vi "CRYClear Main Generator Array.vi"(9 "isMain":bool, 11 "Gen Idx":i32) -> (0 "isMain out":bool)   [LabVIEW 2013]
uses:
  CRYMisc vis settings global.vi
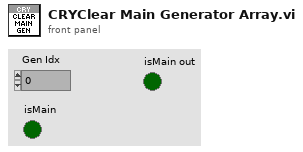
[diagram p1: front panel]
types:
  T1 = cluster{"Gen Idx":i32, "Chn Idx":i32, "Data":sgl[]}[]
  T2 = cluster{"Gen Idx":i32, "Chn Idx":i32, "Data":sgl[]}
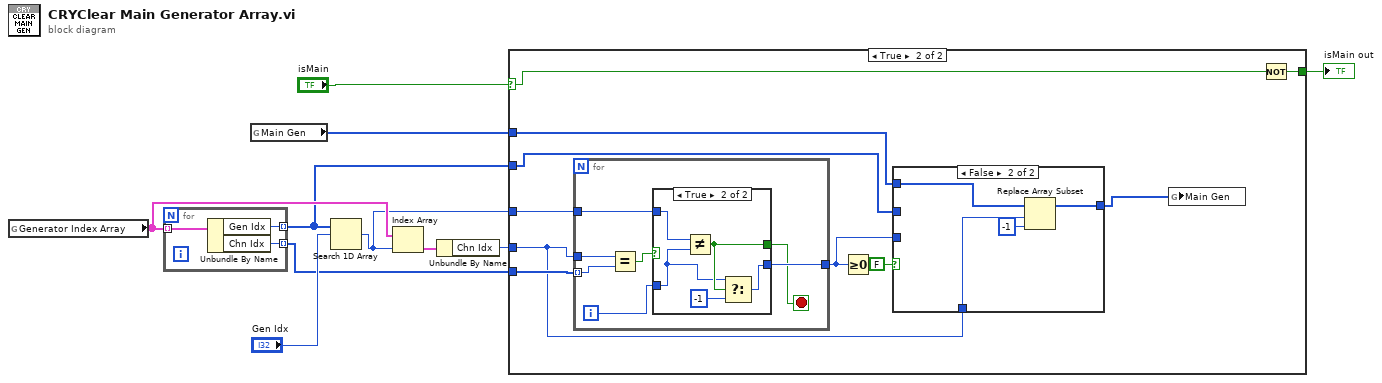
[diagram p0: block diagram]
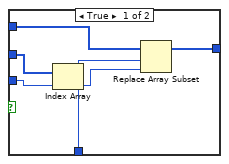
[diagram p3: hidden frame]
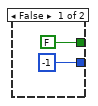
[diagram p4: hidden frame]
diagram:
  n1 = global read "CRYMisc vis settings global.vi" "Generator Index Array"() -> (w9:T1)
  n2 = for {
    tunnel: w9 -> [w13] mode=indexing
    tunnel: [w12] -> w5 mode=indexing
    tunnel: [w11] -> w4 mode=indexing
    n3 = Unbundle By Name(w13) -> ("Gen Idx"=w12:i32, "Chn Idx"=w11:i32)
  }
  n4 = global read "CRYMisc vis settings global.vi" "Main Gen"() -> (w2:i32[])
  n5 = Search 1D Array(1D array=w5, element="Gen Idx") -> (index of element=w3:i32)  [unwired: 1 in]
  n6 = Index Array(array=w9, index=w3) -> (element=w8:T2)
  n7 = Unbundle By Name(w8) -> ("Chn Idx"=w6:i32)
  n8 = case shown="True" "isMain" {
    selector: "isMain" -> [w14 w17]
    tunnel: w6 -> [_ w19]
    tunnel: w5 -> [_ w22]
    tunnel: w4 -> [_ w24]
    tunnel: w3 -> [_ w23]
    tunnel: w2 -> [_ w21]
    tunnel: [w14 w16] -> w1
    frame False {
    }
    frame True {
      n9 = for {
        tunnel: w24 -> [w39] mode=indexing
        tunnel: w19 -> [w41]
        tunnel: w23 -> [w37]
        tunnel: [w36] -> w20
        i -> [w38]
        stop <- w35 stop-if-true
        n10 = Equal?(x=w41, y=w39) -> (x = y?=w40:bool)
        n11 = case shown="True" w40 {
          tunnel: w38 -> [_ w46]
          tunnel: w37 -> [_ w48]
          tunnel: [FALSE w47] -> w35
          tunnel: [-1 w44] -> w36
          frame False {
          }
          frame True {
            n12 = Not Equal?(x=w48, y=w46) -> (x != y?=w47:bool)
            n13 = Select(t=w46, s=w47, f=-1) -> (s? t:f=w44:i32)
          }
        }
      }
      n14 = Greater Or Equal To 0?(x=w20) -> ()  [unwired: 1 out]
      n15 = case shown="False" FALSE {
        tunnel: w22 -> [w30 _]
        tunnel: w21 -> [w28 w34]
        tunnel: w20 -> [w29 _]
        tunnel: w19 -> [w26 w33]
        tunnel: [w25 w32] -> w18
        frame True {
          n16 = Index Array(array=w30, index=w29) -> (element=w27:i32)
          n17 = Replace Array Subset(array=w28, new element=w27, index=w26) -> (w25:i32[])
        }
        frame False {
          n18 = Replace Array Subset(array=w34, new element=-1 ("new element/subarray"), index=w33) -> (w32:i32[])
        }
      }
      n19 = global write "CRYMisc vis settings global.vi" "Main Gen"(w18) -> ()
      n20 = Not(x=w17) -> (.not. x?=w16:bool)
    }
  }
  "isMain out" <- w1
